vi "Flatten Parameters.vi"(0 "Name Space in":refnum<class "Name Space.lvclass">, 1 "Linked List Ref":refnum<data-value>, 5 "Active Unique ID":string, 7 "Indent":i32, 9 "Path":path, 11 "error in (no error)":errorcluster, 12 "Persistence in":refnum<class "IPersist.lvclass">) -> (3 "Linked List Ref out":refnum<data-value>, 4 "Flattened Test Executive":string[](array[string]), 8 "Active Unique ID out":string, 14 "Persistence out":refnum<class "IPersist.lvclass">, 15 "error out":errorcluster)   [LabVIEW 2020, in "Test Executive.lvlib" / "Name Space.lvclass"]
uses:
  <vilib>/gpm_packages/@cs/test-executive/Source/Test Executive/Name Space/Name Space.lvclass
  <vilib>/gpm_packages/@cs/linked-list/Source/Linked List/ILinkedList/ILinked List.lvclass
  <vilib>/gpm_packages/@cs/persistence/source/IPersist/IPersist.lvclass
  <vilib>/gpm_packages/@cs/linked-list/Source/Linked List/Linked List Ref/Linked List Ref.lvclass
  <vilib>/gpm_packages/@cs/linked-list/Source/String Manipulation/String Manipulation.lvlib
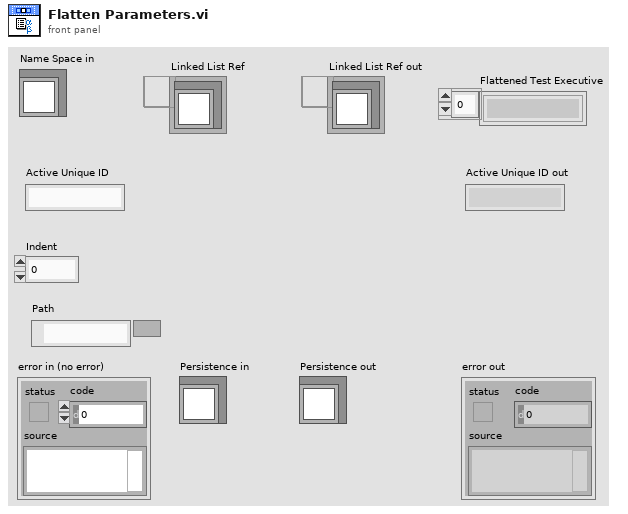
[diagram p1: front panel]
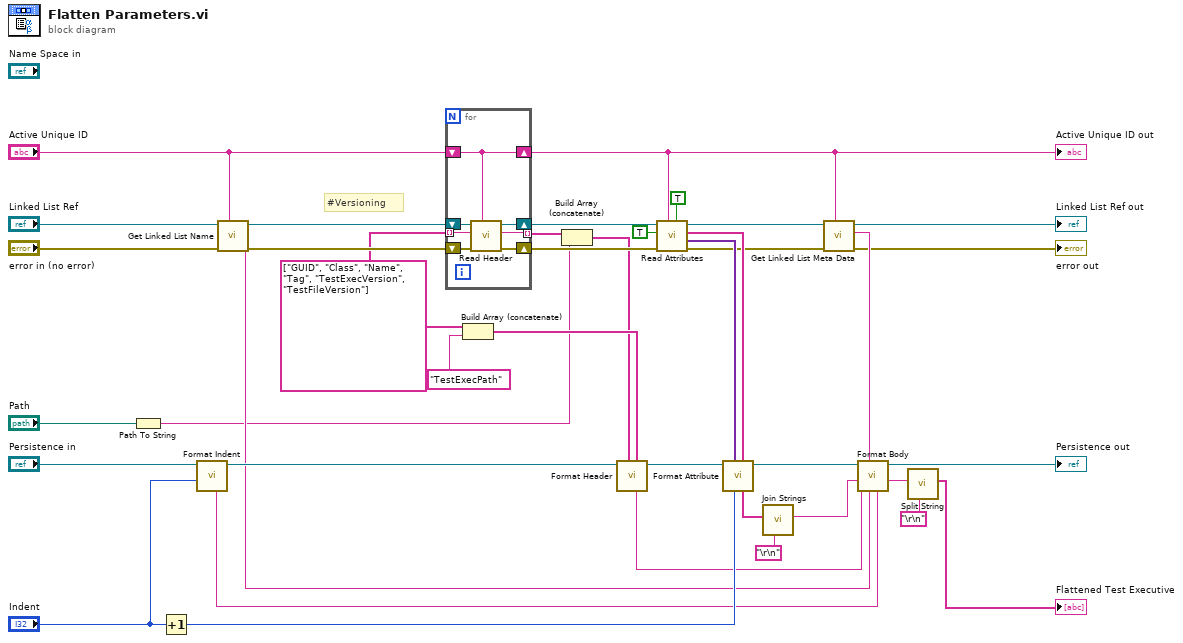
[diagram p0: block diagram]
diagram:
  w6 = string[] ["GUID", "Class", "Name", "Tag", "TestExecVersion", "TestFileVersion"] ("Header Names")
  # "#Versioning"
  n1 = Path To String(path="Path") -> (string=w1:string)
  n2 = Increment(x="Indent") -> (x+1=w29:i32)
  n3 = call-dynamic "Format Indent.vi"("Indent"="Indent", "IPersist in"="Persistence in") -> ("IPersist out"=w38:refnum<class "IPersist.lvclass">, "Indent XML"=w22:string)  [unwired: 7 in, 1 out]
  n4 = call <vilib>:"Get Linked List Name.vi"("Linked List ID"="Active Unique ID", "error in (no error)"="error in (no error)", "Linked List Ref"="Linked List Ref") -> ("error out"=w39:errorcluster, "Linked List Name"=w23:string, "Linked List Ref out"=w40:refnum<data-value>)  [unwired: 5 in, 1 out]
  n5 = for {
    tunnel: w6 -> [w45] mode=indexing
    shift-right: [w46] -> w32
    shift-left: w40 -> [w47]
    tunnel: [w44] -> w2 mode=indexing
    shift-right: [w43] -> w19
    shift-left: "Active Unique ID" -> [w43]
    shift-right: [w41] -> w31
    shift-left: w39 -> [w42]
    n6 = call <vilib>:"Read Header.vi"("Linked List ID"=w43, "error in (no error)"=w42, "Header Name"=w45, "Linked List Ref"=w47) -> ("error out"=w41:errorcluster, "Header Value"=w44:string, "Linked List Ref out"=w46:refnum<data-value>)  [unwired: 4 in, 1 out]
  }
  "Active Unique ID out" <- w19
  n7 = Build Array (concatenate)(w6, "TestExecPath") -> (w5:string[])
  n8 = Build Array (concatenate)(w2, w1) -> (w3:string[])
  n9 = call-dynamic "Format Header.vi"("Name"=w5, "Value"=w3, "IPersist in"=w38) -> ("IPersist out"=w30:refnum<class "IPersist.lvclass">, "Header"=w24:string)  [unwired: 7 in]
  n10 = call <vilib>:"Read Attributes.vi"("Flatten Pointer?"=TRUE, "Linked List ID"=w19, "error in (no error)"=w31, "Include Private?"=TRUE, "Linked List Ref"=w32) -> ("error out"=w8:errorcluster, "Attributes"=w36:variant[], "Attribute Names out"=w35:string[], "Linked List Ref out"=w9:refnum<data-value>)  [unwired: 1 in, 2 out]
  n11 = call-dynamic "Format Attribute.vi"("Attribute Names"=w35, "Indent"=w29, "Attribute Values"=w36, "IPersist in"=w30) -> ("IPersist out"=w10:refnum<class "IPersist.lvclass">, "Attr Strings"=w33:string[])  [unwired: 6 in]
  n12 = call <vilib>:"Join Strings.vi"("Separator (,)"="\r\n", "Strings In"=w33) -> ("String"=w25:string)  [unwired: 9 in]
  n13 = call <vilib>:"Get Linked List Meta Data.vi"("Linked List ID"=w19, "error in (no error)"=w8, "Linked List Ref"=w9) -> ("error out"=→"error out":errorcluster, "Meta Data"=w28:string, "Linked List Ref out"=→"Linked List Ref out":refnum<data-value>)  [unwired: 5 in, 1 out]
  n14 = call-dynamic "Format Body.vi"("Indent"=w22, "Name"=w23, "Meta Data"=w28, "Header"=w24, "Attributes"=w25, "IPersist in"=w10) -> ("String out"=w26:string, "IPersist out"=→"Persistence out":refnum<class "IPersist.lvclass">)  [unwired: 4 in]
  n15 = call <vilib>:"Split String.vi"("Split Pattern"="\r\n", "Input String"=w26) -> ("Split String"=→"Flattened Test Executive":string[])  [unwired: 9 in]
